vi "Set Timed Loop.vi"(11 "CIFCorePlugin in":refnum<class "CIFCorePlugin.lvclass">) -> (1 "Processor":i32, 3 "Priority":i32)   [LabVIEW 2021, in "CIFCorePlugin.lvclass"]
uses:
  CIFCorePlugin.lvclass
  CIFCorePlugin.lvclass/CIFCorePlugin.ctl
  Accessors/Read Common Config.vi
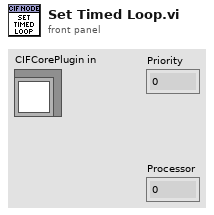
[diagram p1: front panel]
types:
  T1 = typedef "CIFCoreCommon.lvlib/Common Plugin Configuration.ctl" = cluster{"Period (s)":dbl, "Offset (us)":i32, "ClockID":u8, "Priority":i32, "Processor":i32}
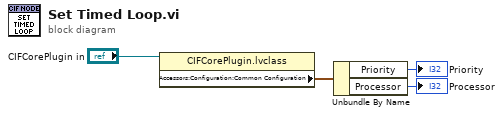
[diagram p0: block diagram]
diagram:
  n1 = property class="CIFCorePlugin.lvclass"(reference="CIFCorePlugin in") -> ("Accessors:Configuration:Common Configuration"=w4:T1)  [unwired: 1 in, 2 out]
  n2 = Unbundle By Name(w4) -> ("Priority"=→"Priority":i32, "Processor"=→"Processor":i32)
